vi "Part Modifier to String.vi"(10 "Pattern Part Modifier":T1) -> (2 "String":string)   [LabVIEW 2020, in "Stream.lvlib" / "URLPattern.lvclass"]
uses:
  URLPattern.lvclass
  Pattern Part Modifier.ctl
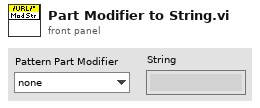
[diagram p1: front panel]
types:
  T1 = typedef "Stream.lvlib/URLPattern.lvclass/Pattern Part Modifier.ctl" = enum16{"none", "optional", "zero-or-more", "one-or-more"}
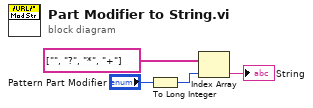
[diagram p0: block diagram]
diagram:
  n1 = To Long Integer(number="Pattern Part Modifier") -> (32bit integer=w1:i32)
  n2 = Index Array(array=string[] ["", "?", "*", "+"], index=w1) -> (element=→"String":string)
